vi "Dialog_AddEditVar.vi"(10 "String in":string, 11 "VariableManagerRef":refnum<vi>) -> (0 "OK?":bool, 2 "Variable Name":string)   [LabVIEW 2013]
doc: "Dialog for adding/editing variables from the SetList table. The dialog is pre-populated from \"String In.\"\nIf user types in an existing variable name, any changes will overwrite the existing variable. De-slecting the \"overwrite?\" checkbox will re-populate the existing values.\nThis dialog uses the Variable Manager checks to ensure all variables are well-formed, prompting the user for necessary changes."
uses:
  VariableManagerCodes/VariableManager/VariableManager.lvclass
  VariableManagerCodes/Variable/Variable.lvclass
  VariableManagerCodes/API/VariableManagerAPI.lvlib
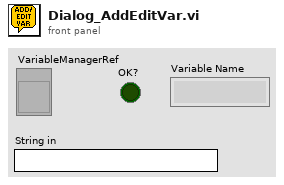
[diagram p1: front panel]
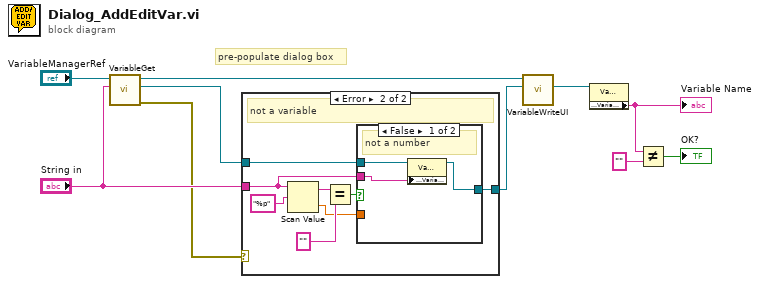
[diagram p0: block diagram]
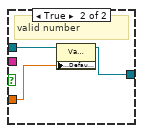
[diagram p3: hidden frame]
diagram:
  # "pre-populate dialog box"
  n1 = call "VariableGet.vi"("VariableName"="String in", "VariableManagerRef in"="VariableManagerRef") -> ("error out"=w8:errorcluster, "Variable"=w7:refnum<class "Variable.lvclass">, "VariableManagerRef out"=w6:refnum<vi>)  [unwired: 7 in]
  n2 = case shown="Error" w8 {
    tunnel: w7 -> [w11 w14]
    tunnel: [w11 w13] -> w5
    tunnel: "String in" -> [_ w12]
    frame No Error {
      # "variable exists!"
    }
    frame Error {
      # "not a variable"
      n3 = Scan Value(string=w12, format string="%p") -> (output string=w18:string, value=w15:dbl)  [unwired: 1 in]
      n4 = Equal?(x=w18, y="") -> (x = y?=w16:bool)
      n5 = case shown="False" w16 {
        tunnel: w15 -> [_ w23]
        tunnel: w14 -> [w22 w25]
        tunnel: [w21 w24] -> w13
        tunnel: w12 -> [w20 _]
        frame False {
          # "not a number"
          n6 = property class="Variable.lvclass"(reference=w22, "Accessors:VariableName"=w20) -> (reference out=w21:refnum<class "Variable.lvclass">)  [unwired: 1 in, 1 out]
        }
        frame True {
          # "valid number"
          n7 = property class="Variable.lvclass"(reference=w25, "Accessors:DefaultValue"=w23) -> (reference out=w24:refnum<class "Variable.lvclass">)  [unwired: 1 in, 1 out]
        }
      }
    }
  }
  n8 = call "VariableWriteUI.vi"("VariableFill"=w5, "VariableManagerRef in"=w6) -> ("VariableWrote"=w4:refnum<class "Variable.lvclass">)  [unwired: 8 in, 1 out]
  n9 = property class="Variable.lvclass"(reference=w4) -> ("Accessors:VariableName"=w1:string)  [unwired: 1 in, 2 out]
  "Variable Name" <- w1
  n10 = Not Equal?(x=w1, y="") -> (x != y?=→"OK?":bool)
